vi "Config.vi"(8 "error in (no error)":errorcluster, 10 "Setting":variant, 11 "Lambda Gen Plus":refnum<class "Lambda Gen Plus.lvclass">) -> (0 "error out":errorcluster, 3 "Lambda Gen Plus out":refnum<class "Lambda Gen Plus.lvclass">)   [LabVIEW 2025, in "Power Supply.lvlib" / "Lambda Gen Plus.lvclass"]
uses:
  Lambda Gen Plus.lvclass
  Lambda Gen Plus.lvclass/Lambda Gen Plus.ctl
  <instrlib>/TDK-Lambda G Series/TDK-Lambda G Series.lvlib
  PS Channel/Power Supply Channel.lvclass
  PS Channel configuration/Power Supply Channel configuration.lvclass
  Users/Public/Documents/Sandia National Labs/TSS Plugin/Abstract Engine.lvlibp/Plugin/Abstract/Abstract Instrument/Channel.ctl
  Users/Public/Documents/Sandia National Labs/TSS Plugin/Abstract Engine.lvlibp/Plugin/Abstract/Abstract Instrument/Abstract Instrument.lvclass
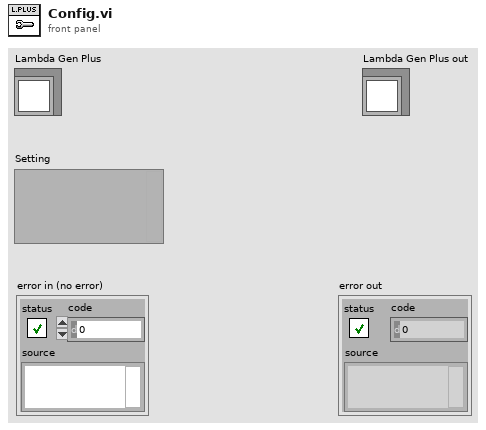
[diagram p1: front panel]
types:
  T1 = typedef "Abstract Engine.lvlibp/Abstract Instrument.lvclass/Channel.ctl" = cluster{"Alias":string, "DataType":enum16{"Anaolg Input", "Waveform"}, "Unit":enum16{"---", "V", "A", "Ohm", "Hz", "uF", "degC", "deg"}, "Upper limit":dbl, "Lower limit":dbl, "Measurement":variant}
  T2 = typedef "Abstract Engine.lvlibp/Channel configuration.lvclass/Default Channel.ctl" = cluster{"Address":string, "SW Alias":string, "Enabled":bool, "Type":string, "Description":string}
  T3 = typedef "Power Supply.lvlib/Power Supply Channel configuration.lvclass/PS Channel Setting.ctl" = cluster{"Driver":string, "Pin":string, "Test Voltage":string, "Voltage Low":dbl, "Voltage Norminal":dbl, "Voltage High":dbl, "PreTest Voltage":dbl, "PreTest Current":dbl, "Current Limit":dbl}
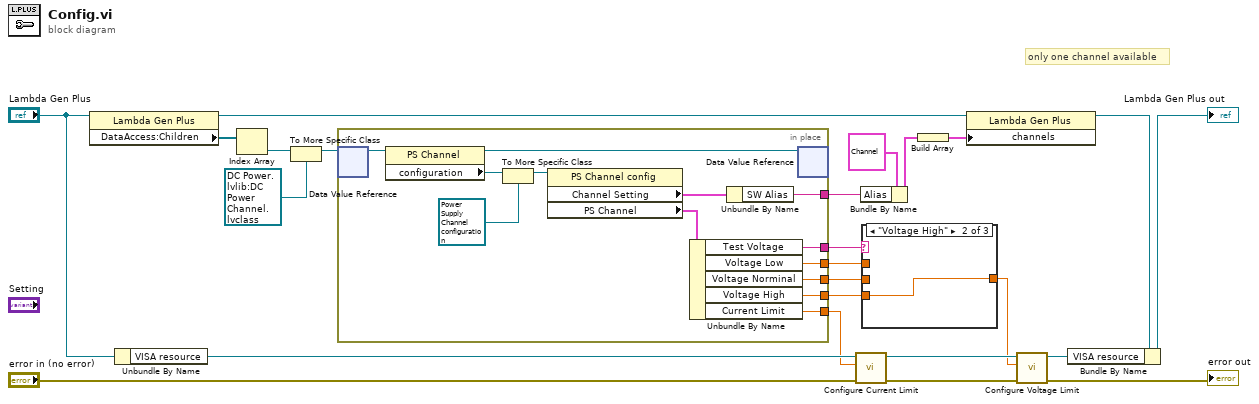
[diagram p0: block diagram]
diagram:
  # "only one channel available"
  n1 = property class="Lambda Gen Plus"(reference="Lambda Gen Plus") -> (reference out=w15:refnum<class "Lambda Gen Plus.lvclass">, "DataAccess:Children"=w16:refnum<data-value>[])  [unwired: 1 in, 1 out]
  n2 = Unbundle By Name("Lambda Gen Plus") -> ("VISA resource"=w23:refnum<visa-resource-name>)
  n3 = Index Array(array=w16) -> (element=w17:refnum<data-value>)  [unwired: 1 in]
  n4 = To More Specific Class(target class=refnum<data-value> refnum ("data value reference"), reference=w17) -> (specific class reference=w18:refnum<data-value>)  [unwired: 1 in, 1 out]
  n5 = in-place {
    in-place-border: [w30] -> w9
    in-place-border: [w29] -> w8
    in-place-border: [w28] -> w7
    in-place-border: [w27] -> w6
    in-place-border: [w26] -> w5
    in-place-border: [w25] -> w4
    # "Initialize the front panel controls when loaded"
    n6 = in-place-dvr #1(w18) -> (w37:refnum<class "Power Supply Channel.lvclass">)  [unwired: 1 out]
    n7 = property class="PS Channel"(reference=w37) -> (reference out=w36:refnum<class "Power Supply Channel.lvclass">, "configuration"=w35:refnum<class "CEF_serializable configuration.lvclass">)  [unwired: 1 in, 1 out]
    n8 = To More Specific Class(target class=refnum<class "Power Supply Channel configuration.lvclass"> refnum ("DC Power.lvlib:DCPower Channel configuration.lvclass"), reference=w35) -> (specific class reference=w34:refnum<class "Power Supply Channel configuration.lvclass">)  [unwired: 1 in, 1 out]
    n9 = property class="PS Channel config"(reference=w34) -> ("Channel Setting"=w32:T2, "PS Channel"=w31:T3)  [unwired: 1 in, 2 out]
    n10 = Unbundle By Name(w31) -> ("Test Voltage"=w28:string, "Voltage Low"=w27:dbl, "Voltage Norminal"=w26:dbl, "Voltage High"=w25:dbl, "Current Limit"=w29:dbl)
    n11 = Unbundle By Name(w32) -> ("SW Alias"=w30:string)
    n12 = in-place-dvr #1(w36) -> ()  [unwired: 2 out]
  }
  n13 = call <instrlib>:"Configure Current Limit.vi"("error in (no error)"="error in (no error)", "Current Limit (0A)"=w8, "VISA resource name"=w23) -> ("error out"=w22:errorcluster, "VISA resource name out"=w21:refnum<visa-resource-name>)  [unwired: 7 in]
  n14 = Bundle By Name(cluster=T1 {"Alias"="ch0", "DataType"=enum."Anaolg Input", "Unit"=enum."V", "Upper limit"=10.0, "Lower limit"=-10.0, "Measurement"=variant} ("Channel"), "Alias"=w9) -> (w10:T1)
  n15 = case shown="\"Voltage High\"" w7 {
    tunnel: w6 -> [_ _ w40]
    tunnel: w5 -> [w38 _ _]
    tunnel: w4 -> [_ w39 _]
    tunnel: [w38 w39 w40] -> w3
    frame "Voltage Norminal", Default {
    }
    frame "Voltage High" {
    }
    frame "Voltage Low" {
    }
  }
  n16 = Build Array(w10) -> (w2:T1[])
  n17 = property class="Lambda Gen Plus"(reference=w15, "channels"=w2) -> (reference out=w11:refnum<class "Lambda Gen Plus.lvclass">)  [unwired: 1 in, 1 out]
  n18 = call <instrlib>:"Configure Voltage Limit.vi"("error in (no error)"=w22, "Voltage Limit (0V)"=w3, "VISA resource name"=w21) -> ("error out"=→"error out":errorcluster, "VISA resource name out"=w20:refnum<visa-resource-name>)  [unwired: 7 in]
  n19 = Bundle By Name(cluster=w11, "VISA resource"=w20) -> (→"Lambda Gen Plus out":refnum<class "Lambda Gen Plus.lvclass">)
